vi "SpinningDisCShutter.vi"(8 "error in (no error)":errorcluster, 10 "Ring":u16(ring) items=["Open", "Close"]) -> (0 "error out":errorcluster)   [LabVIEW 2015]
panel:
  out "return count":u32
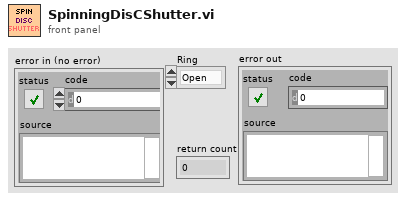
[diagram p1: front panel]
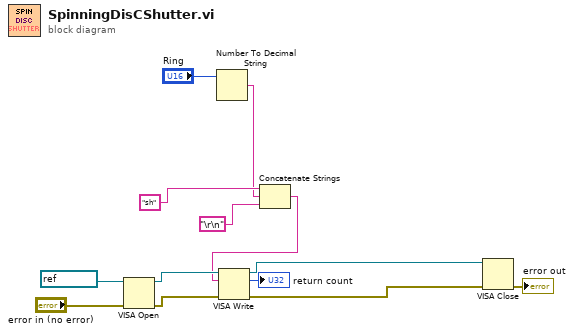
[diagram p0: block diagram]
diagram:
  n1 = VISA Open(error in (no error)="error in (no error)", VISA resource name=refnum<visa-resource-name> "COM1") -> (VISA resource name=w10:refnum<visa-resource-name>, error out=w11:errorcluster)  [unwired: 3 in]
  n2 = Number To Decimal String(number="Ring") -> (decimal integer string=w1:string)  [unwired: 1 in]
  n3 = Concatenate Strings("sh", w1, "\r\n") -> (w8:string)
  n4 = VISA Write(VISA resource name=w10, write buffer=w8, error in (no error)=w11) -> (VISA resource name out=w6:refnum<visa-resource-name>, return count=→"return count":u32, error out=w5:errorcluster)
  n5 = VISA Close(VISA resource name=w6, error in (no error)=w5) -> (error out=→"error out":errorcluster)
